vi "Read Time.vi"(11 "Simple Actor in":refnum<class "Simple Actor.lvclass">) -> (2 "Time":dbl)   [LabVIEW 2017, in "Simple Actor.lvlib" / "Simple Actor.lvclass"]
uses:
  Simple Actor.lvclass
  Simple Actor.lvclass/Simple Actor.ctl
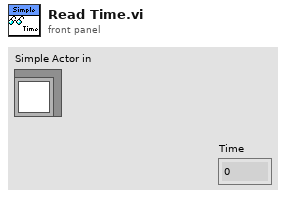
[diagram p1: front panel]
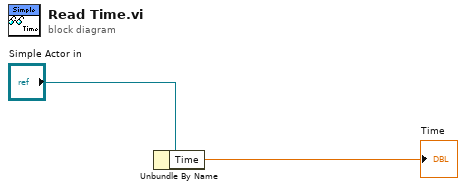
[diagram p0: block diagram]
diagram:
  n1 = Unbundle By Name("Simple Actor in") -> ("Time"=→"Time":dbl)
